vi "DSF.Execution.Runtime.Plugin Manager.Get Plugins Folder.vi"(8 "error in (no error)":errorcluster, 11 "Plugin Manager in":refnum<class "Plugin Manager.lvclass">) -> (0 "error out":errorcluster, 2 "Plugins folder":path, 3 "Plugin Manager out":refnum<class "Plugin Manager.lvclass">)   [LabVIEW 2016, in "DSF.Engine.lvlib" / "Plugin Manager.lvclass"]
uses:
  Plugin Manager.lvclass
  Plugin Manager.lvclass/Plugin Manager.ctl
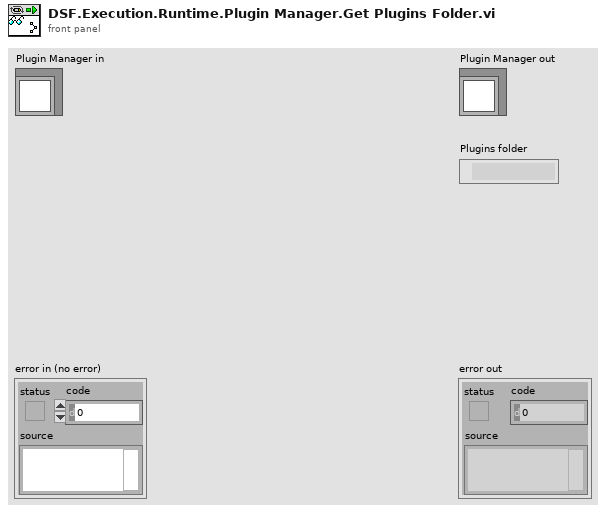
[diagram p1: front panel]
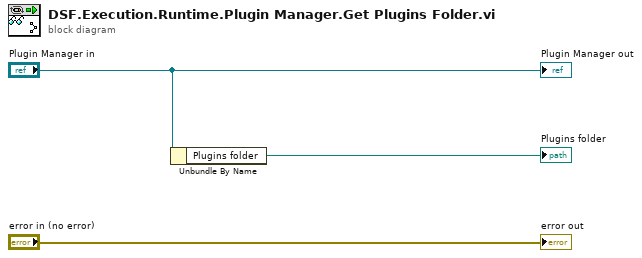
[diagram p0: block diagram]
diagram:
  n1 = Unbundle By Name("Plugin Manager in") -> ("Plugins folder"=→"Plugins folder":path)
  "error out" <- "error in (no error)"
  "Plugin Manager out" <- "Plugin Manager in"
